vi "Test Basic Function 4.vi"() -> ()   [LabVIEW 2014]
uses:
  <vilib>/Aledyne-TSXperts/Arduino Compatible Compiler for LabVIEW/addons/Arduino Math/Arduino Math.lvlib
panel:
  out "result 5":sgl
  out "sin(x) 2":sgl
  out "result 4":sgl
  out "result 3":sgl
  out "floor(x)":sgl
  out "sin(x)":sgl
  out "result 2":sgl
  out "ceil(x)":sgl
  out "atan2(y, x)":sgl
  out "atan(x)":sgl
  out "asin(x)":sgl
  out "result":sgl
  out "Error Out":errorcluster
  in  "Error In":errorcluster
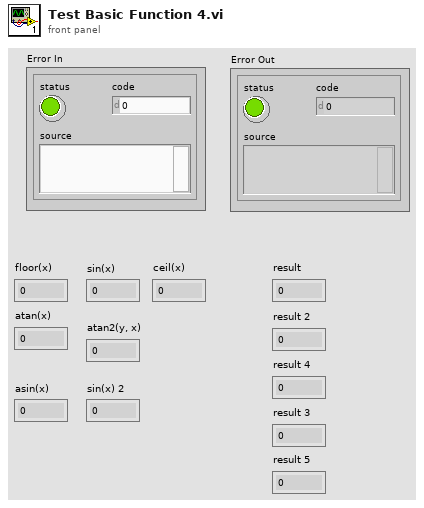
[diagram p1: front panel]
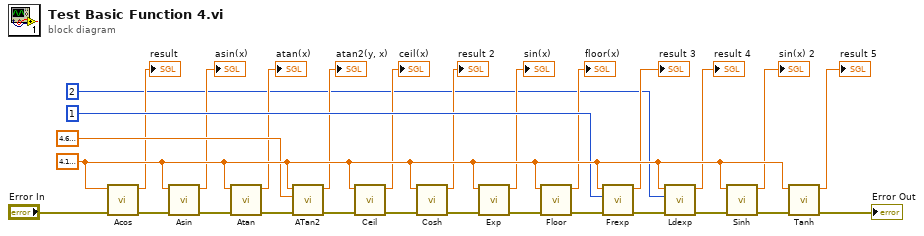
[diagram p0: block diagram]
diagram:
  w28 = sgl 4.2 ("x")
  n1 = call <vilib>:"Acos.vi"("Error In"="Error In", "x"=w28) -> ("Error Out"=w26:errorcluster, "result"=→"result":sgl)  [unwired: 8 in]
  n2 = call <vilib>:"Asin.vi"("Error In"=w26, "x"=w28) -> ("Error Out"=w25:errorcluster, "asin(x)"=→"asin(x)":sgl)  [unwired: 8 in]
  n3 = call <vilib>:"Atan.vi"("Error In"=w25, "x"=w28) -> ("Error Out"=w24:errorcluster, "atan(x)"=→"atan(x)":sgl)  [unwired: 8 in]
  n4 = call <vilib>:"ATan2.vi"("Error In"=w24, "y"=sgl 4.7 ("x"), "x"=w28) -> ("Error Out"=w23:errorcluster, "atan2(y, x)"=→"atan2(y, x)":sgl)  [unwired: 7 in]
  n5 = call <vilib>:"Ceil.vi"("Error In"=w23, "x"=w28) -> ("Error Out"=w22:errorcluster, "ceil(x)"=→"ceil(x)":sgl)  [unwired: 8 in]
  n6 = call <vilib>:"Cosh.vi"("Error In"=w22, "x"=w28) -> ("Error Out"=w21:errorcluster, "result"=→"result 2":sgl)  [unwired: 8 in]
  n7 = call <vilib>:"Exp.vi"("Error In"=w21, "x"=w28) -> ("Error Out"=w20:errorcluster, "sin(x)"=→"sin(x)":sgl)  [unwired: 8 in]
  n8 = call <vilib>:"Floor.vi"("Error In"=w20, "x"=w28) -> ("Error Out"=w19:errorcluster, "floor(x)"=→"floor(x)":sgl)  [unwired: 8 in]
  n9 = call <vilib>:"Frexp.vi"("Error In"=w19, "pexp"=u32 1, "x"=w28) -> ("Error Out"=w18:errorcluster, "result"=→"result 3":sgl)  [unwired: 7 in]
  n10 = call <vilib>:"Ldexp.vi"("Error In"=w18, "pexp"=i16 2, "x"=w28) -> ("Error Out"=w17:errorcluster, "result"=→"result 4":sgl)  [unwired: 7 in]
  n11 = call <vilib>:"Sinh.vi"("Error In"=w17, "x"=w28) -> ("Error Out"=w16:errorcluster, "sin(x)"=→"sin(x) 2":sgl)  [unwired: 8 in]
  n12 = call <vilib>:"Tanh.vi"("Error In"=w16, "x"=w28) -> ("Error Out"=→"Error Out":errorcluster, "result"=→"result 5":sgl)  [unwired: 8 in]
